vi "UNLOADING_DOOR_PLC.vi"(0 "Unloading cyc Data":T1) -> (3 "all rows":string[][](array[string]), 4 "DOOR NO.":string, 6 "QR Code":string, 8 "Unloading cyc Data 2":T1)   [LabVIEW 2017]
uses:
  Controls/Feed_Cyc_Data.ctl
  Controls/Unloading_Cyc_Data.ctl
  <vilib>/Utility/file.llb/Read Delimited Spreadsheet (string).vi
  <vilib>/Utility/file.llb/Write Delimited Spreadsheet (string).vi
panel:
  in  "error in":errorcluster
  out "error out":errorcluster
  out "?":T2
  in  "Enum":enum16{"FEED", "LOADED"}(ring)=enum."LOADED"
  in  "Door No":i32
  out "output array":string[][](array[string])
  out "error out":errorcluster
  in  "error in (no error)":errorcluster
  in  "?":T2
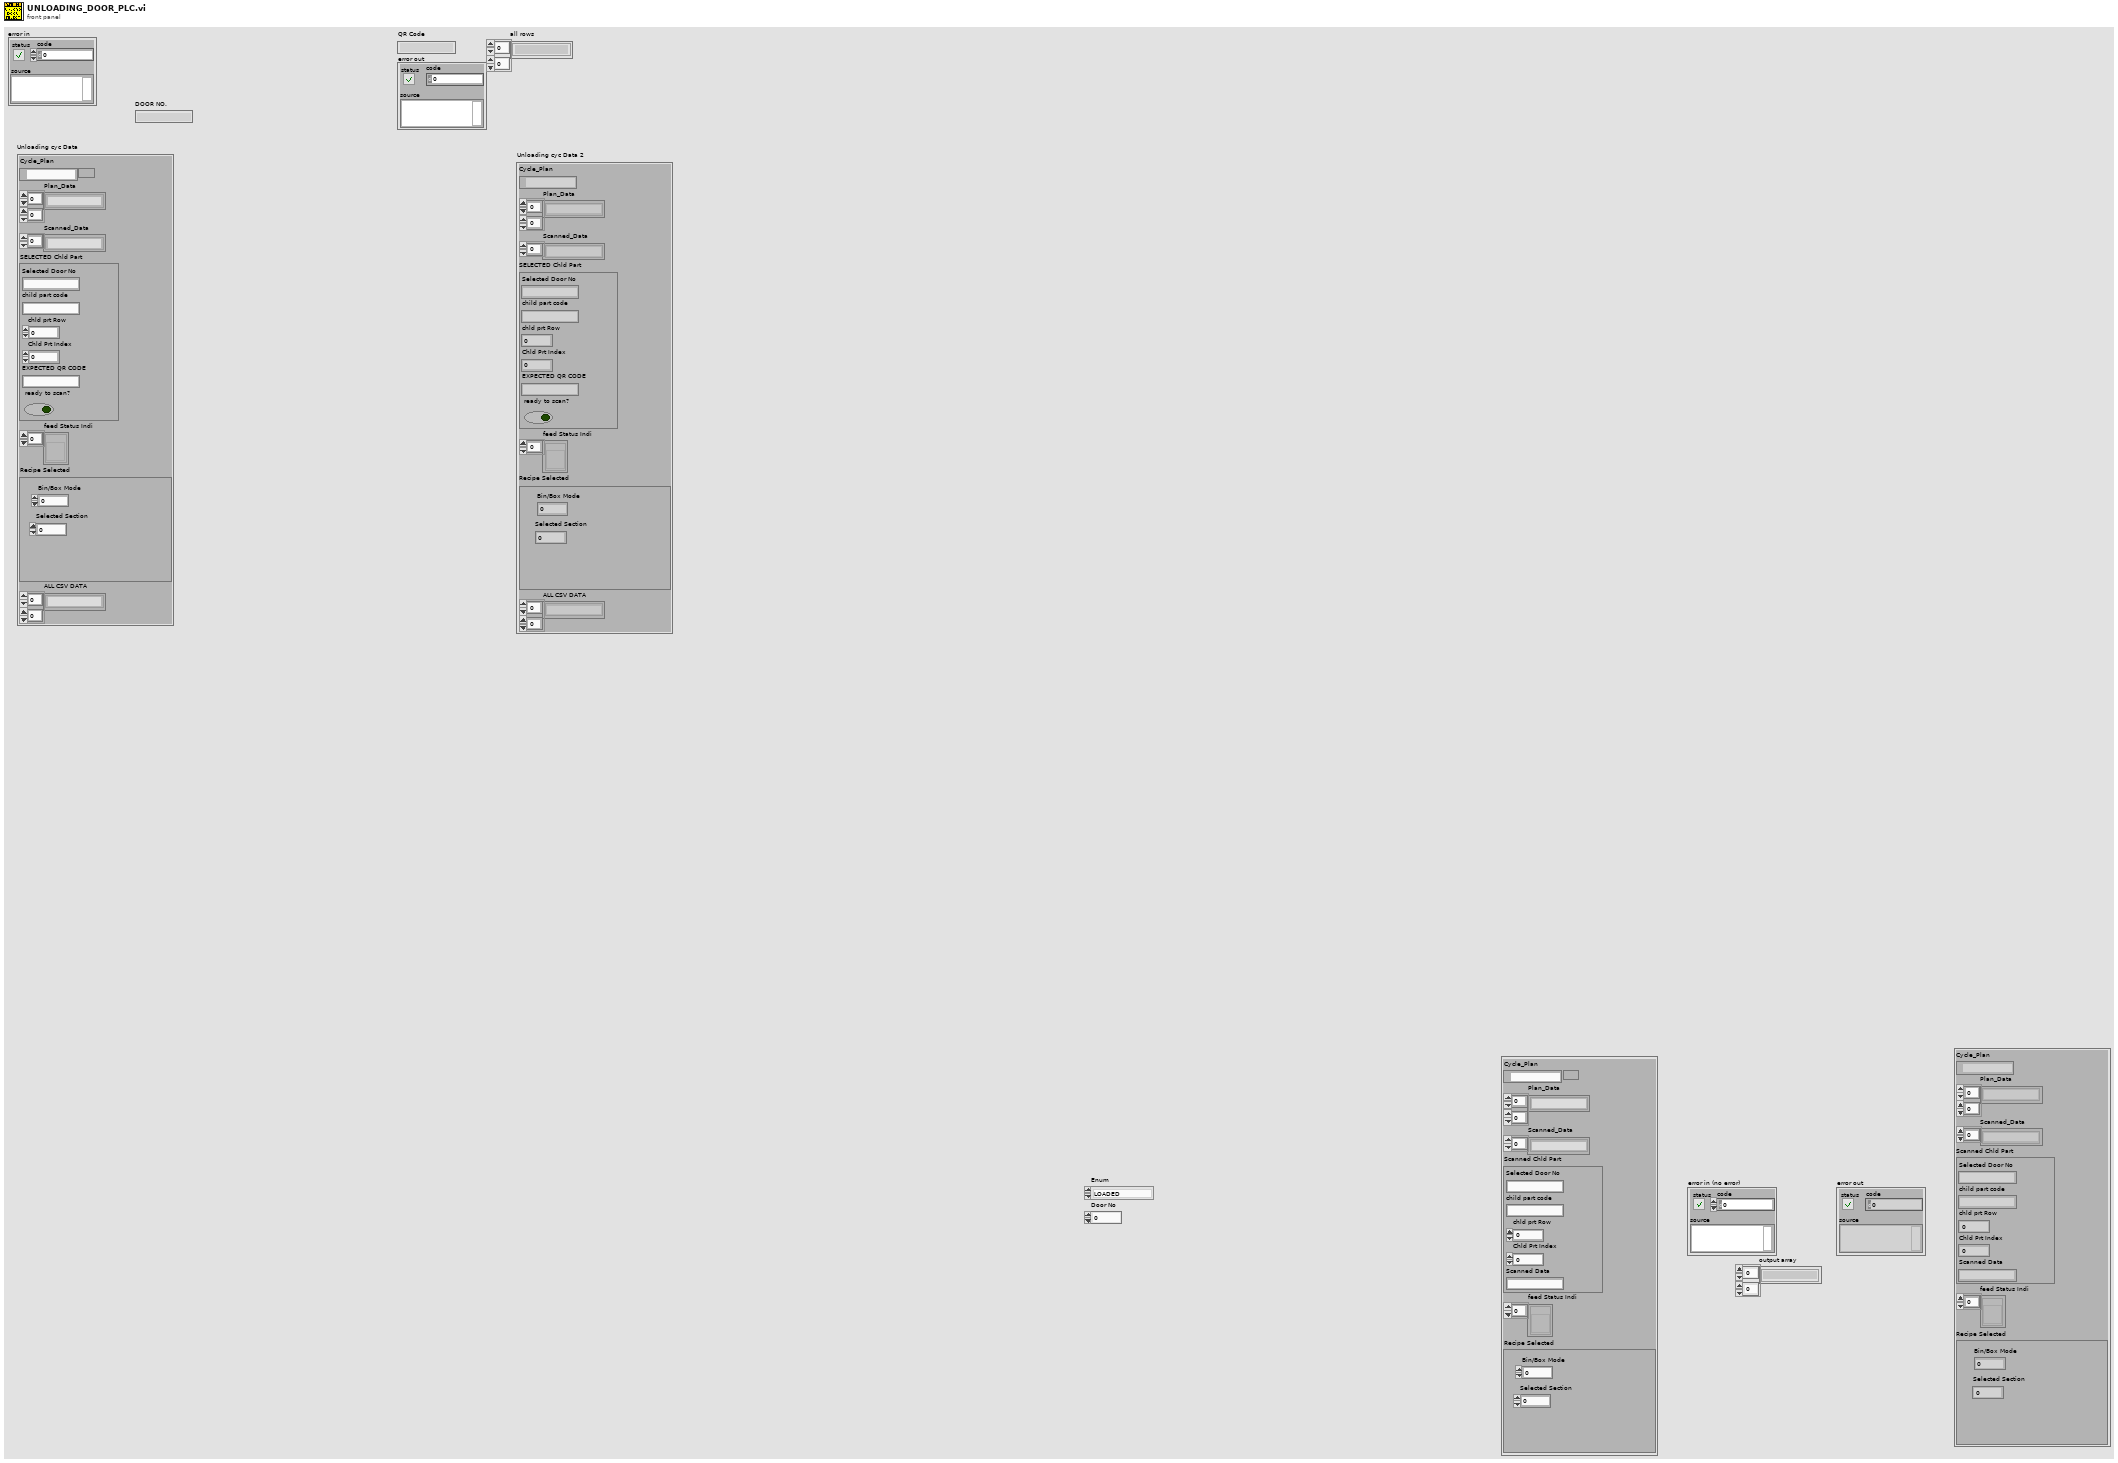
[diagram p1: front panel]
types:
  T1 = typedef "Unloading_Cyc_Data.ctl" = cluster{"Cycle_Plan":path, "Plan_Data":string[][], "Scanned_Data":string[], "SELECTED Chld Part":cluster{"Selected Door No":string, "child part code":string, "chld prt Row":i32, "Chld Prt Index":i32, "EXPECTED QR CODE":string, "ready to scan?":bool}, "feed Status Indi":refnum<vi>[], "Recipe Selected":cluster{"Bin/Box Mode":i32, "Selected Section":i32}, "ALL CSV DATA":string[][]}
  T2 = typedef "Feed_Cyc_Data.ctl" = cluster{"Cycle_Plan":path, "Plan_Data":string[][], "Scanned_Data":string[], "Scanned Chld Part":cluster{"Selected Door No":string, "child part code":string, "chld prt Row":i32, "Chld Prt Index":i32, "Scanned Data":string}, "feed Status Indi":refnum<vi>[], "Recipe Selected":cluster{"Bin/Box Mode":i32, "Selected Section":i32}}
  T3 = cluster{"Selected Door No":string, "child part code":string, "chld prt Row":i32, "Chld Prt Index":i32, "Scanned Data":string}
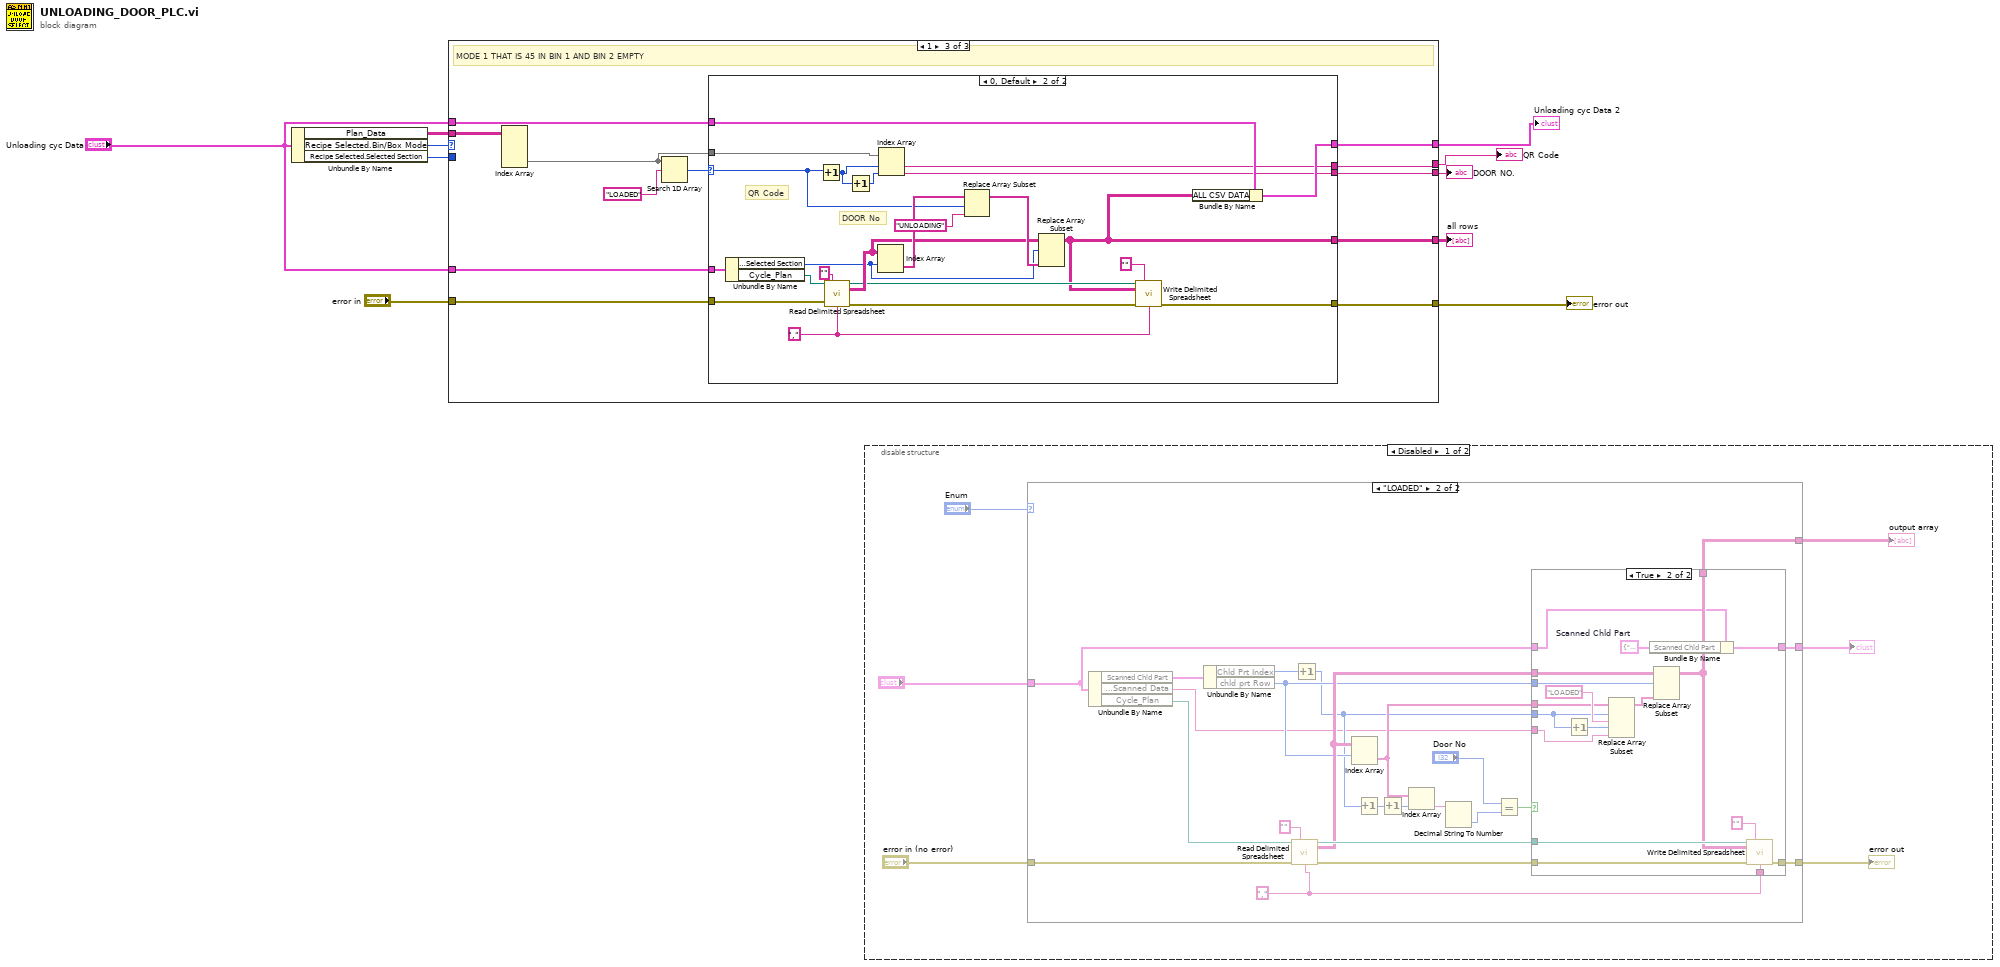
[diagram p0: block diagram]
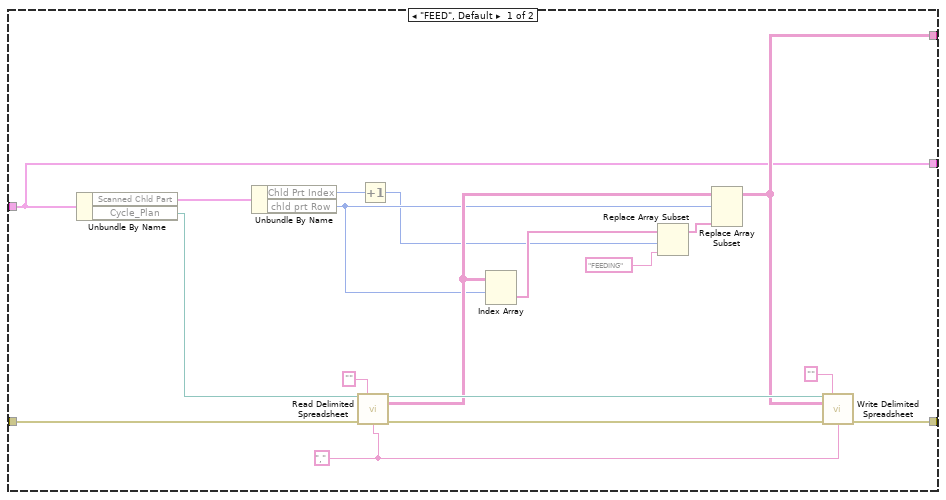
[diagram p2: hidden frame]
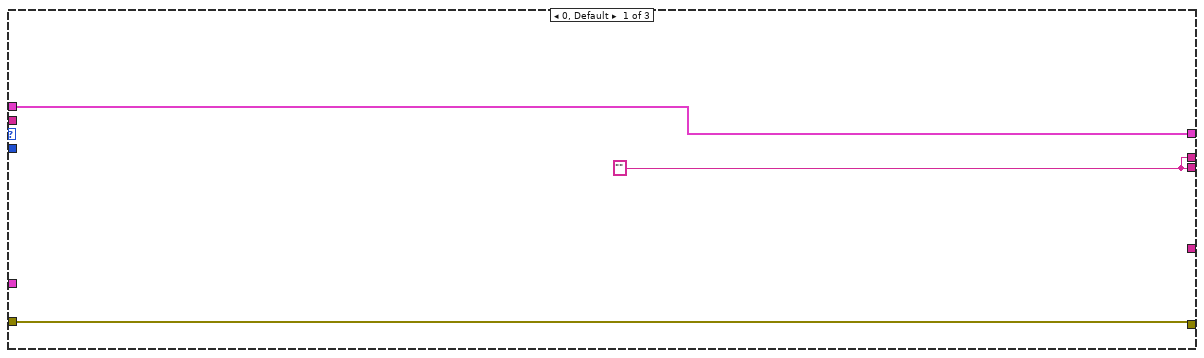
[diagram p5: hidden frame]
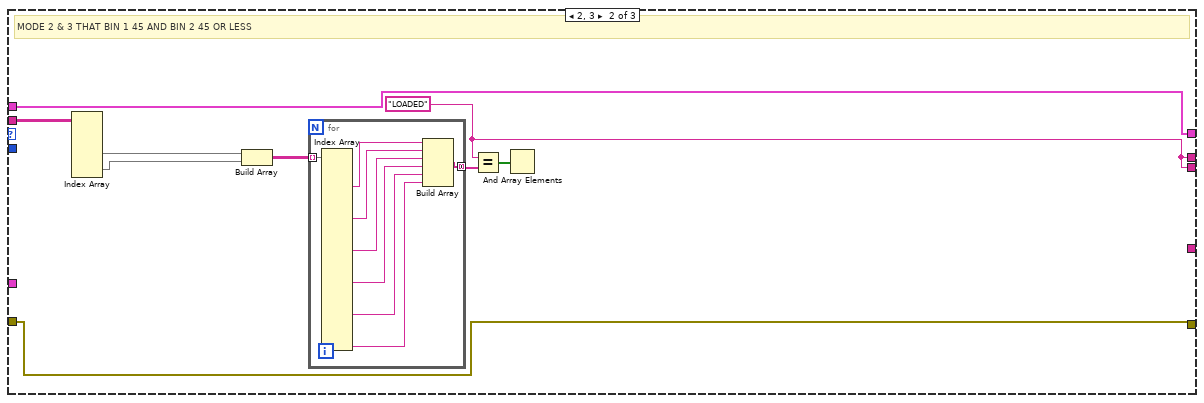
[diagram p6: hidden frame]
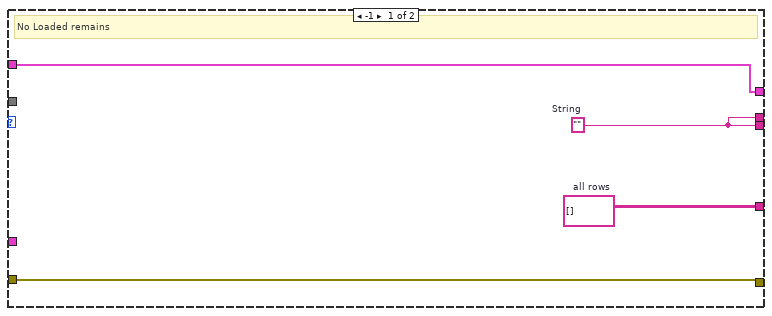
[diagram p7: hidden frame]
diagram:
  n1 = Unbundle By Name("Unloading cyc Data") -> ("Plan_Data"=w9:string[][], "Recipe Selected.Bin/Box Mode"=w8:i32, "Recipe Selected.Selected Section"=w6:i32)
  n2 = case shown="1" w8 {
    tunnel: w9 -> [_ w22 w42]
    tunnel: [w13 w16 w41] -> w10
    tunnel: [w13 w16 w40] -> w7
    tunnel: w6 -> [_ _ _]
    tunnel: "Unloading cyc Data" -> [_ _ w39]
    tunnel: "error in" -> [w12 w15 w38]
    tunnel: [w12 w15 w37] -> w4
    tunnel: [_ _ w36] -> w3
    tunnel: "Unloading cyc Data" -> [w11 w14 w32]
    tunnel: [w11 w14 w31] -> w1
    frame 0, Default {
      w13 = ""
    }
    frame 2, 3 {
      w16 = "LOADED"
      # "MODE 2 & 3 THAT BIN 1 45 AND BIN 2 45 OR LESS"
      n3 = Index Array(array=w22) -> (element #2=w21:string[], element #3=w20:string[])  [unwired: 6 in, 1 out]
      n4 = Build Array(w21, w20) -> (w19:string[][])
      n5 = for {
        tunnel: w19 -> [w30] mode=indexing
        tunnel: [w23] -> w18 mode=concatenating
        n6 = Index Array(array=w30) -> (element #3=w29:string, element #7=w28:string, element #11=w27:string, element #15=w26:string, element #19=w25:string, element #23=w24:string)  [unwired: 23 in, 17 out]
        n7 = Build Array(w29, w28, w27, w26, w25, w24) -> (w23:string[])
      }
      n8 = Equal?(x=w16, y=w18) -> (x = y?=w17:bool[])
      n9 = And Array Elements(Boolean array=w17) -> ()  [unwired: 1 out]
    }
    frame 1 {
      # "MODE 1 THAT IS 45 IN BIN 1 AND BIN 2 EMPTY"
      n10 = Index Array(array=w42) -> (element #2=w35:string[])  [unwired: 4 in, 1 out]
      n11 = Search 1D Array(1D array=w35, element="LOADED") -> (index of element=w33:i32)  [unwired: 1 in]
      n12 = case shown="0, Default" w33 {
        selector: w33 -> [_ w58]
        tunnel: [w46 w48] -> w41
        tunnel: w35 -> [_ w69]
        tunnel: [w46 w47] -> w40
        tunnel: w39 -> [_ w66]
        tunnel: w38 -> [w45 w63]
        tunnel: [w45 w55] -> w37
        tunnel: [w44 w50] -> w36
        tunnel: w32 -> [w43 w51]
        tunnel: [w43 w49] -> w31
        frame -1 {
          w44 = string[][] []  # all rows
          w46 = ""  # String
          # "No Loaded remains"
        }
        frame 0, Default {
          w53 = ","
          # "QR Code"
          # "DOOR No"
          n13 = Unbundle By Name(w66) -> ("Recipe Selected.Selected Section"=w52:i32, "Cycle_Plan"=w64:path)
          n14 = Increment(x=w58) -> (x+1=w67:i32)
          n15 = call-poly <vilib>:"Read Delimited Spreadsheet.vi"("file path (dialog if empty)"=w64, "format (%s)"="", "error in (no error)"=w63, "delimiter (\\t)"=w53) -> ("new file path (Not A Path if cancelled)"=w54:path, "all rows"=w59:string[][], "error out"=w56:errorcluster)  [unwired: 6 in, 3 out]
          n16 = Increment(x=w67) -> (x+1=w68:i32)
          n17 = Index Array(array=w59, index (row)=w52) -> (element=w61:string[])  [unwired: 1 in]
          n18 = Index Array(array=w69, index #1=w67, index #2=w68) -> (element #1=w47:string, element #2=w48:string)
          n19 = Replace Array Subset(array=w61, new element="UNLOADING", index=w58) -> (w60:string[])
          n20 = Replace Array Subset(array=w59, new element=w60, index (row)=w52) -> (w50:string[][])  [unwired: 1 in]
          n21 = call-poly <vilib>:"Write Delimited Spreadsheet.vi"("file path (dialog if empty)"=w54, "format (%s)"="", "2D data"=w50, "error in (no error)"=w56, "delimiter (\\t)"=w53) -> ("error out"=w55:errorcluster)  [unwired: 9 in, 1 out]
          n22 = Bundle By Name(cluster=w51, "ALL CSV DATA"=w50) -> (w49:T1)
        }
      }
    }
  }
  "DOOR NO." <- w10
  "QR Code" <- w7
  "error out" <- w4
  "all rows" <- w3
  "Unloading cyc Data 2" <- w1
  n23 = disable-structure shown="Disabled" {
    frame Disabled {
      n24 = case shown="\"LOADED\"" "Enum" {
        tunnel: "?" -> [w76 w97]
        tunnel: "error in (no error)" -> [w90 w114]
        tunnel: [w89 w113] -> w73
        tunnel: [w80 w109] -> w72
        tunnel: [w76 w96] -> w70
        frame "FEED", Default {
          w79 = ","
          n25 = Unbundle By Name(w76) -> ("Scanned Chld Part"=w88:T3, "Cycle_Plan"=w92:path)
          n26 = Unbundle By Name(w88) -> ("Chld Prt Index"=w84:i32, "chld prt Row"=w86:i32)
          n27 = call-poly <vilib>:"Read Delimited Spreadsheet.vi"("file path (dialog if empty)"=w92, "format (%s)"="", "error in (no error)"=w90, "delimiter (\\t)"=w79) -> ("new file path (Not A Path if cancelled)"=w91:path, "all rows"=w87:string[][], "error out"=w93:errorcluster)  [unwired: 6 in, 3 out]
          n28 = Increment(x=w84) -> (x+1=w83:i32)
          n29 = Index Array(array=w87, index (row)=w86) -> (element=w85:string[])  [unwired: 1 in]
          n30 = Replace Array Subset(array=w85, new element="FEEDING", index=w83) -> (w81:string[])
          n31 = Replace Array Subset(array=w87, new element=w81, index (row)=w86) -> (w80:string[][])  [unwired: 1 in]
          n32 = call-poly <vilib>:"Write Delimited Spreadsheet.vi"("file path (dialog if empty)"=w91, "format (%s)"="", "2D data"=w80, "error in (no error)"=w93, "delimiter (\\t)"=w79) -> ("error out"=w89:errorcluster)  [unwired: 9 in, 1 out]
        }
        frame "LOADED" {
          w108 = ","
          n33 = Unbundle By Name(w97) -> ("Scanned Chld Part"=w112:T3, "Scanned Chld Part.Scanned Data"=w95:string, "Cycle_Plan"=w94:path)
          n34 = Unbundle By Name(w112) -> ("Chld Prt Index"=w110:i32, "chld prt Row"=w106:i32)
          n35 = call-poly <vilib>:"Read Delimited Spreadsheet.vi"("file path (dialog if empty)"=w94, "format (%s)"="", "error in (no error)"=w114, "delimiter (\\t)"=w108) -> ("new file path (Not A Path if cancelled)"=w115:path, "all rows"=w111:string[][], "error out"=w116:errorcluster)  [unwired: 6 in, 3 out]
          n36 = Increment(x=w110) -> (x+1=w104:i32)
          n37 = Index Array(array=w111, index (row)=w106) -> (element=w105:string[])  [unwired: 1 in]
          n38 = Increment(x=w104) -> (x+1=w102:i32)
          n39 = Increment(x=w102) -> (x+1=w103:i32)
          n40 = Index Array(array=w105, index=w103) -> (element=w101:string)
          n41 = Decimal String To Number(string=w101) -> (number=w100:i32)  [unwired: 2 in, 1 out]
          n42 = Equal?(x="Door No", y=w100) -> (x = y?=w98:bool)
          n43 = case shown="True" w98 {
            tunnel: w116 -> [w118 w136]
            tunnel: w115 -> [_ w135]
            tunnel: [w118 w134] -> w113
            tunnel: w111 -> [w119 w133]
            tunnel: [w119 w130] -> w109
            tunnel: w108 -> [_ w129]
            tunnel: w106 -> [_ w128]
            tunnel: w105 -> [_ w127]
            tunnel: w104 -> [_ w121]
            tunnel: w97 -> [w117 w125]
            tunnel: [w117 w124] -> w96
            tunnel: w95 -> [_ w120]
            frame False {
            }
            frame True {
              w123 = T3 {"Selected Door No"="", "child part code"="", "chld prt Row"=0, "Chld Prt Index"=0, "Scanned Data"=""}  # Scanned Chld Part
              n44 = Increment(x=w121) -> (x+1=w122:i32)
              n45 = Replace Array Subset(array=w127, new element #1="LOADED", index #1=w121, new element #2=w120, index #2=w122) -> (w131:string[])
              n46 = Bundle By Name(cluster=w125, "Scanned Chld Part"=w123) -> (w124:T2)
              n47 = Replace Array Subset(array=w133, new element=w131, index (row)=w128) -> (w130:string[][])  [unwired: 1 in]
              n48 = call-poly <vilib>:"Write Delimited Spreadsheet.vi"("file path (dialog if empty)"=w135, "format (%s)"="", "2D data"=w130, "error in (no error)"=w136, "delimiter (\\t)"=w129) -> ("error out"=w134:errorcluster)  [unwired: 9 in, 1 out]
            }
          }
        }
      }
      "error out" <- w73
      "output array" <- w72
      "?" <- w70
    }
    frame Enabled {
    }
  }
